vi "Interpolation Solver.vi"() -> ()   [LabVIEW 2023]
doc: "Demonstrates different types of interpolation on a set of raw data. The types of interpolation demonstrated in this example are Linear, Polynomial, Spline, and Rational."
uses:
  <vilib>/Analysis/NI_AALPro.lvlib
panel:
  in  "Tab Control":enum32{"Graph", "Data"}(tab)
  out "Raw and Interpolated Data":T1(graph)
  in  "Original Data (X,Y)":dbl[][](array[numeric])=[[0.0, 1.0], [1.2, 2.700000047683716], [2.0, 7.400000095367432], [3.0, 150.0], [3.5, 140.0], [4.0, 80.0], [5.0, 220.0]] format="%0.2f"
  out "Interpolated Data (X,Y)":dbl[][](array[numeric]) format="%0.2f"
  in  "Stop":bool
  in  "Interpolation factor (n)":i32(slide)=4 scale=0.0..20.0
  in  "Type of Interpolation":T2(ring)=enum."Spline"
  # "Overview: Demonstrates different types of interpolation on a set of raw data.\nRequirements: LabVIEW Full Development System\nInstructions: \n1. Run the VI.\n2. Change the Type of Interpolation and Interpolation factor (n) and verify how it affects the results displayed on the Graph and Data tabs.\n3. Click Stop to stop the VI."
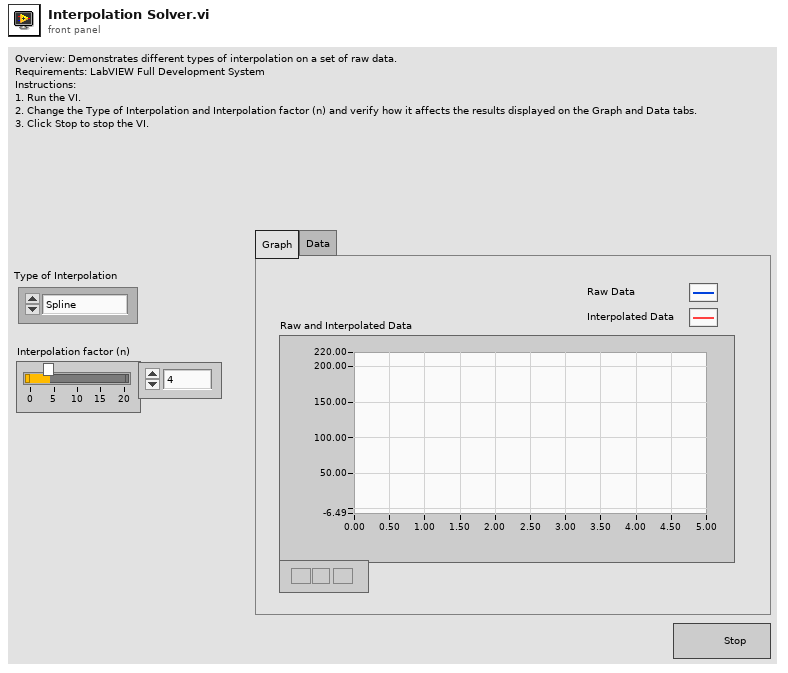
[diagram p1: front panel]
types:
  T1 = cluster{"Original Data (X,Y)":dbl[], "Original Data (X,Y)":dbl[]}[]
  T2 = enum16{"Linear", "Polynomial", "Spline", "Rational"}
  T3 = cluster{"Original Data (X,Y)":dbl[], "Original Data (X,Y)":dbl[]}
  T4 = typedef "NI_Matrix.lvlib/RealMatrix.ctl" = dbl[][]
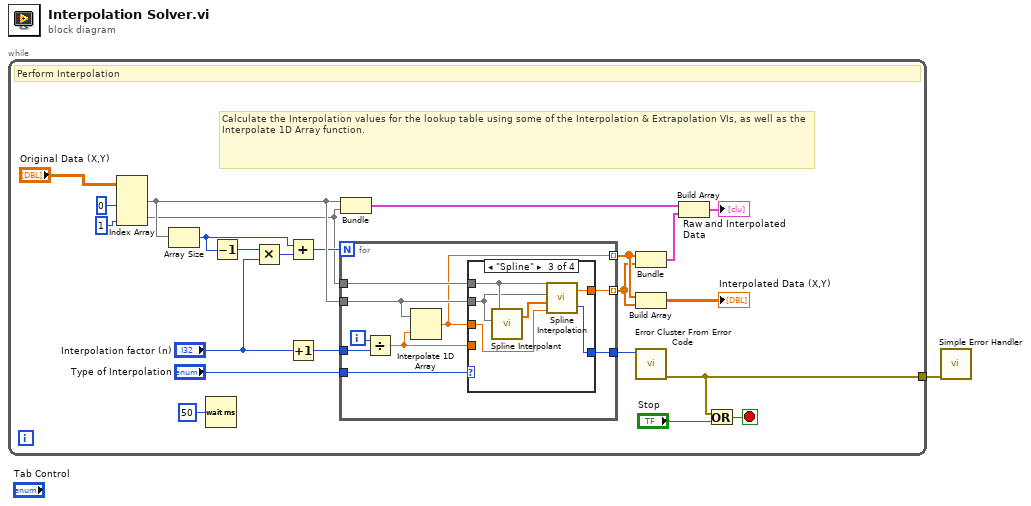
[diagram p0: block diagram]
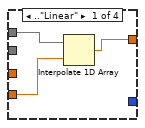
[diagram p2: hidden frame]
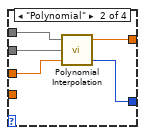
[diagram p3: hidden frame]
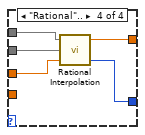
[diagram p4: hidden frame]
diagram:
  n1 = while {
    tunnel: [w5] -> w1
    stop <- w6 stop-if-true
    # "Calculate the Interpolation values for the lookup table using some of the Interpolation & Extrapolation VIs, as well as the Interpolate 1D Array function."
    # "Perform Interpolation"
    n2 = Index Array(array="Original Data (X,Y)", index (col) #1=0, index (col) #2=1 ("index (col)")) -> (element #1=w16:dbl[], element #2=w8:dbl[])  [unwired: 2 in]
    n3 = Array Size(array=w16) -> (size(s)=w12:i32)
    n4 = Wait (ms)(milliseconds to wait=u32 50) -> ()  [unwired: 1 out]
    n5 = Decrement(x=w12) -> (x-1=w15:i32)
    n6 = Multiply(x=w15, y="Interpolation factor (n)") -> (x*y=w13:i32)
    n7 = Add(x=w12, y=w13) -> (x+y=w11:i32)
    n8 = Increment(x="Interpolation factor (n)") -> (x+1=w14:i32)
    n9 = for {
      N: w11 -> [_]
      tunnel: w8 -> [w33]
      tunnel: w16 -> [w27]
      tunnel: [w32] -> w7
      tunnel: "Type of Interpolation" -> [w28]
      tunnel: w14 -> [w30]
      tunnel: [w29] -> w3 mode=indexing
      tunnel: [w26] -> w4 mode=indexing
      i -> [w31]
      n10 = Divide(x=w31, y=w30) -> (x/y=w25:dbl)
      n11 = Interpolate 1D Array(1:w25, 2:w27) -> (0:w26:dbl)
      n12 = case shown="\"Spline\"" w28 {
        tunnel: w26 -> [_ w41 w44 w48]
        tunnel: [w35 w40 w42 w50] -> w29
        tunnel: [_ w39 w43 w49] -> w32
        tunnel: w27 -> [_ w38 w45 w51]
        tunnel: w33 -> [w36 w37 w47 w52]
        tunnel: w25 -> [w34 _ _ _]
        frame .."Linear" {
          n13 = Interpolate 1D Array(1:w34, 2:w36) -> (0:w35:dbl)
        }
        frame "Polynomial" {
          n14 = call <vilib>:"Polynomial Interpolation.vi"("x value"=w41, "X"=w38, "Y"=w37) -> ("error"=w39:i32, "interpolation value"=w40:dbl)  [unwired: 1 out]
        }
        frame "Spline" {
          n15 = call <vilib>:"Spline Interpolant.vi"("X"=w45, "Y"=w47) -> ("Interpolant"=w46:dbl[])  [unwired: 2 in, 1 out]
          n16 = call <vilib>:"Spline Interpolation.vi"("x value"=w44, "Interpolant"=w46, "X"=w45, "Y"=w47) -> ("error"=w43:i32, "interpolation value"=w42:dbl)
        }
        frame "Rational".. {
          n17 = call <vilib>:"Rational Interpolation.vi"("x value"=w48, "X"=w51, "Y"=w52) -> ("error"=w49:i32, "interpolation value"=w50:dbl)  [unwired: 1 out]
        }
      }
    }
    n18 = Bundle("Original Data (X,Y)"=w16, "Original Data (X,Y)"=w8) -> (w17:T3)  [unwired: 1 in]
    n19 = Bundle(w4, w3) -> (w19:cluster{dbl[], dbl[]})  [unwired: 1 in]
    n20 = Build Array(w4, w3) -> (→"Interpolated Data (X,Y)":T4)
    n21 = call <vilib>:"Error Cluster From Error Code.vi"("error code (0)"=w7) -> ("error out"=w5:errorcluster)  [unwired: 8 in]
    n22 = Build Array(w17, w19) -> (→"Raw and Interpolated Data":T1)
    n23 = Or(x=w5, y="Stop") -> (x .or. y?=w6:bool)
  }
  n24 = call <vilib>:"Simple Error Handler.vi"("error in (no error)"=w1) -> ()  [unwired: 4 in, 5 out]
